vi "Sub_SaveXLSX.vi"(0 "y_var":dbl[][](array[numeric]), 1 "x_var":dbl[][](array[numeric]), 2 "Validity":i32[](array[numeric]), 3 "DirPath":path) -> ()   [LabVIEW 2014]
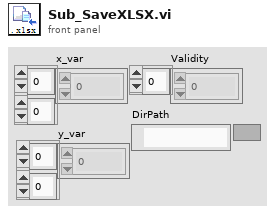
[diagram p1: front panel]
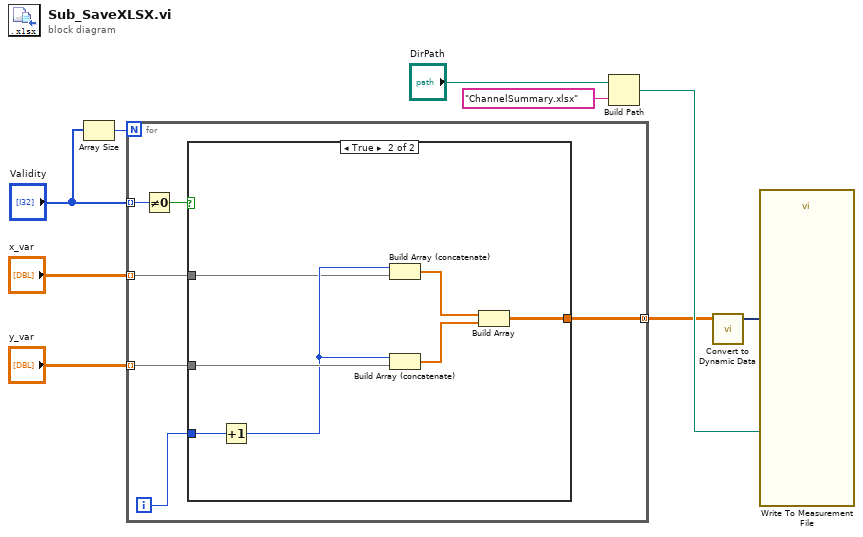
[diagram p0: block diagram]
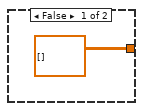
[diagram p2: hidden frame]
diagram:
  n1 = Array Size(array="Validity") -> (size(s)=w9:i32)
  n2 = for {
    N: w9 -> [_]
    tunnel: "Validity" -> [w15] mode=indexing
    tunnel: "x_var" -> [w12] mode=indexing
    tunnel: "y_var" -> [w11] mode=indexing
    tunnel: [w10] -> w2 mode=concatenating
    i -> [w13]
    n3 = Not Equal To 0?(x=w15) -> (x != 0?=w14:bool)
    n4 = case shown="True" w14 {
      tunnel: w13 -> [_ w23]
      tunnel: w12 -> [_ w20]
      tunnel: w11 -> [_ w22]
      tunnel: [dbl[][] [] w17] -> w10
      frame False {
      }
      frame True {
        n5 = Increment(x=w23) -> (x+1=w21:i32)
        n6 = Build Array (concatenate)(w21, w20) -> (w18:dbl[])
        n7 = Build Array (concatenate)(w21, w22) -> (w19:dbl[])
        n8 = Build Array(w18, w19) -> (w17:dbl[][])
      }
    }
  }
  n9 = Build Path(base path="DirPath", name or relative path="ChannelSummary.xlsx") -> (appended path=w3:path)
  n10 = call "Convert to Dynamic Data"("2D Array"=w2) -> ("Dynamic Data Type"=w1:dynamicdata)  [unwired: 3 in]
  n11 = call "Write To Measurement File"("Signals"=w1, "Filename"=w3) -> ()  [unwired: 15 in, 3 out]
